vi "Low-speed-warn.vi"(11 "Boolean":bool) -> (3 "Airspeed Warning Indicator":string)   [LabVIEW 2025]
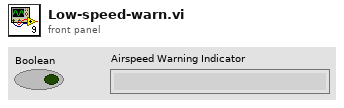
[diagram p1: front panel]
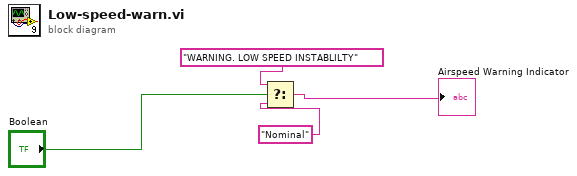
[diagram p0: block diagram]
diagram:
  n1 = Select(t="WARNING. LOW SPEED INSTABLILTY", s="Boolean", f="Nominal") -> (s? t:f=→"Airspeed Warning Indicator":string)
